vi "Main.vi"() -> ()   [LabVIEW 2017, in "AbstractFactoryPatternDemo.lvclass"]
uses:
  AbstractFactoryPatternDemo.lvclass
  FactoryProducer Class/FactoryProducer.lvclass
  ConsoleOut/Print Options.ctl
  AbstractFactory Class/AbstractFactory.lvclass
  afShape Class/afShape.lvclass
  afColor Class/afColor.lvclass
panel:
  out "error out":errorcluster
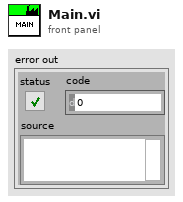
[diagram p1: front panel]
types:
  T1 = typedef "Print Options.ctl" = enum16{"Create", "Get Reference", "Print", "Print Header", "Close"}
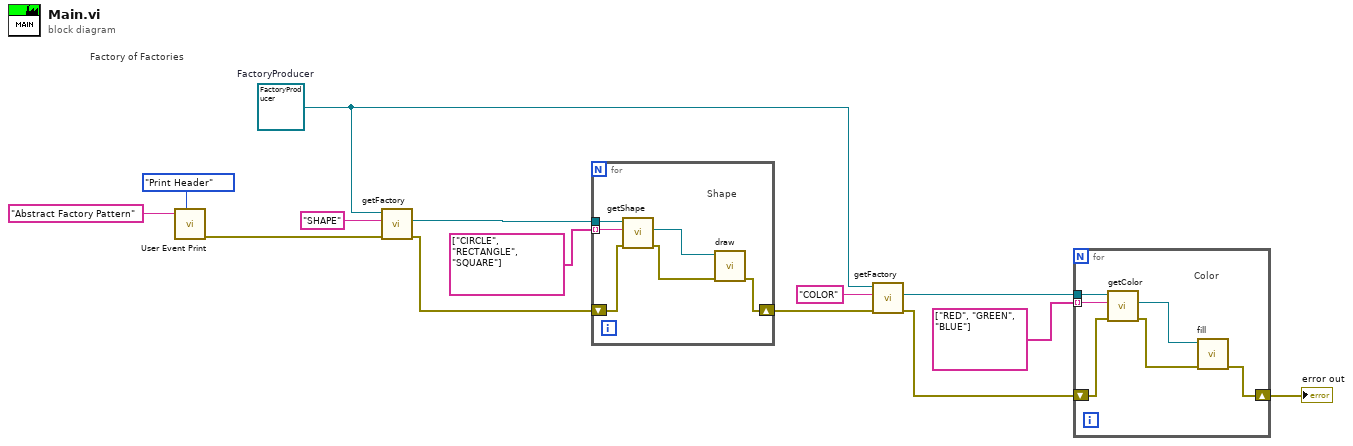
[diagram p0: block diagram]
diagram:
  w1 = refnum<class "FactoryProducer.lvclass"> refnum  # FactoryProducer
  # "Factory of Factories"
  n1 = call "User Event Print.vi"("Options"=Print_Options."Print Header", "String to Print"="Abstract Factory Pattern") -> ("error out"=w7:errorcluster)  [unwired: 8 in, 1 out]
  n2 = call "getFactory.vi"("error in (no error)"=w7, "choice"="SHAPE", "FactoryProducer in"=w1) -> ("error out"=w12:errorcluster, "AbstractFactory"=w13:refnum<class "AbstractFactory.lvclass">)  [unwired: 6 in, 1 out]
  n3 = for {
    tunnel: w13 -> [w20]
    tunnel: string[] ["CIRCLE", "RECTANGLE", "SQUARE"] ("Shape") -> [w16] mode=indexing
    shift-right: [w15] -> w2
    shift-left: w12 -> [w17]
    # "Shape"
    n4 = call-dynamic "getShape.vi"("error in (no error)"=w17, "Shape"=w16, "AbstractFactory in"=w20) -> ("error out"=w19:errorcluster, "afShape.lvclass"=w18:refnum<class "afShape.lvclass">)  [unwired: 6 in, 1 out]
    n5 = call-dynamic "draw.vi"("error in (no error)"=w19, "afShape in"=w18) -> ("error out"=w15:errorcluster)  [unwired: 8 in, 1 out]
  }
  n6 = call "getFactory.vi"("error in (no error)"=w2, "choice"="COLOR", "FactoryProducer in"=w1) -> ("error out"=w11:errorcluster, "AbstractFactory"=w10:refnum<class "AbstractFactory.lvclass">)  [unwired: 6 in, 1 out]
  n7 = for {
    tunnel: w10 -> [w23]
    tunnel: string[] ["RED", "GREEN", "BLUE"] ("Shape") -> [w22] mode=indexing
    shift-right: [w21] -> w3
    shift-left: w11 -> [w26]
    # "Color"
    n8 = call-dynamic "getColor.vi"("error in (no error)"=w26, "Color"=w22, "AbstractFactory in"=w23) -> ("error out"=w24:errorcluster, "afColor.lvclass"=w25:refnum<class "afColor.lvclass">)  [unwired: 6 in, 1 out]
    n9 = call-dynamic "fill.vi"("error in (no error)"=w24, "afColor in"=w25) -> ("error out"=w21:errorcluster)  [unwired: 8 in, 1 out]
  }
  "error out" <- w3
